vi "Register Data Handling.vi"(6 "VolatusAPI in":refnum<class "VolatusAPI.lvclass">, 8 "error in (no error)":errorcluster, 11 "LocalGraphBuffer in":refnum<class "LocalGraphBuffer.lvclass">) -> (0 "error out":errorcluster, 3 "LocalGraphBuffer out":refnum<class "LocalGraphBuffer.lvclass">)   [LabVIEW 2020, in "VolatusGUIElements.lvlib" / "LocalGraphBuffer.lvclass"]
uses:
  LocalGraphBuffer.lvclass
  C:/dev/lv20CE/relink/lv-vecto/Vecto/SubscribedDataHandler/SubscribedDataHandler.lvclass
  Volatus/VolatusAPI/VolatusAPI.lvclass
  LocalGraphBuffer.lvclass/LocalGraphBuffer.ctl
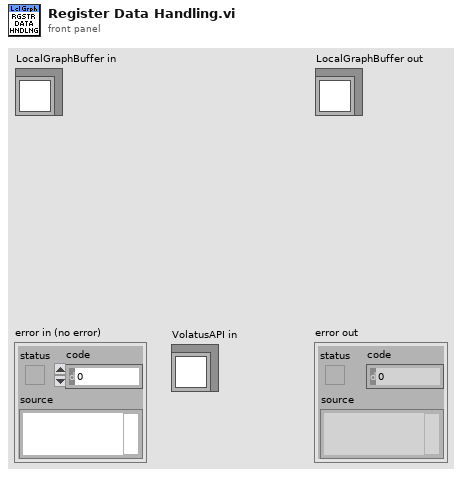
[diagram p1: front panel]
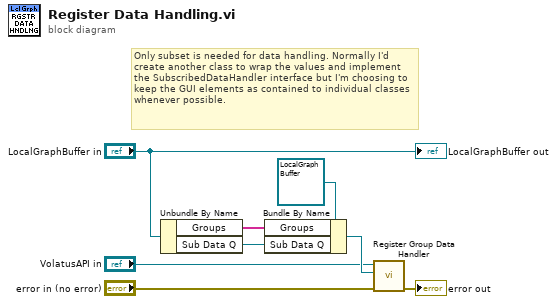
[diagram p0: block diagram]
diagram:
  # "Only subset is needed for data handling. Normally I'd create another class to wrap the values and implement the SubscribedDataHandler interface but I'm choosing to keep the GUI elements as contained to individual classes whenever possible."
  n1 = Unbundle By Name("LocalGraphBuffer in") -> ("Groups"=w1:string[], "Sub Data Q"=w6:refnum<queue>)
  n2 = Bundle By Name(cluster=refnum<class "LocalGraphBuffer.lvclass"> refnum ("LocalGraphBuffer in"), "Groups"=w1, "Sub Data Q"=w6) -> (w5:refnum<class "LocalGraphBuffer.lvclass">)
  n3 = call "Register Group Data Handler.vi"("error in (no error)"="error in (no error)", "Data Handler"=w5, "VolatusAPI in"="VolatusAPI in") -> ("error out"=→"error out":errorcluster)  [unwired: 7 in, 1 out]
  "LocalGraphBuffer out" <- "LocalGraphBuffer in"
